vi "Ex_1a.vi"() -> ()   [LabVIEW 2023]
uses:
  <vilib>/platform/TimedLoop/XDataNode/XDataNode.xnode
  <vilib>/Platform/TimedLoop/XDataNode/nitl_modes.ctl
  <vilib>/Platform/TimedLoop/XDataNode/wakeup.ctl
  <vilib>/Platform/TimedLoop/XDataNode/timing_clust.ctl
  <vilib>/DAQmx/create/channels.llb/DAQmx Create Channel (AI-Voltage-Basic).vi
  <vilib>/DAQmx/read.llb/DAQmx Read (Analog DBL 1Chan 1Samp).vi
  <vilib>/Analysis/NI_AALBase.lvlib
  <vilib>/Analysis/baseanly.llb/Mean (DBL).vi
panel:
  out "min":dbl
  out "max":dbl
  out "mean":dbl
  out "Current  Value":dbl
  out "Waveform Graph":dynamicdata(graph)
  in  "Acceleration Unit 2":bool
  out "Current Data Point":dbl
  out "Waveform Chart":dbl(graph)
  in  "?":bool
  in  "?":bool
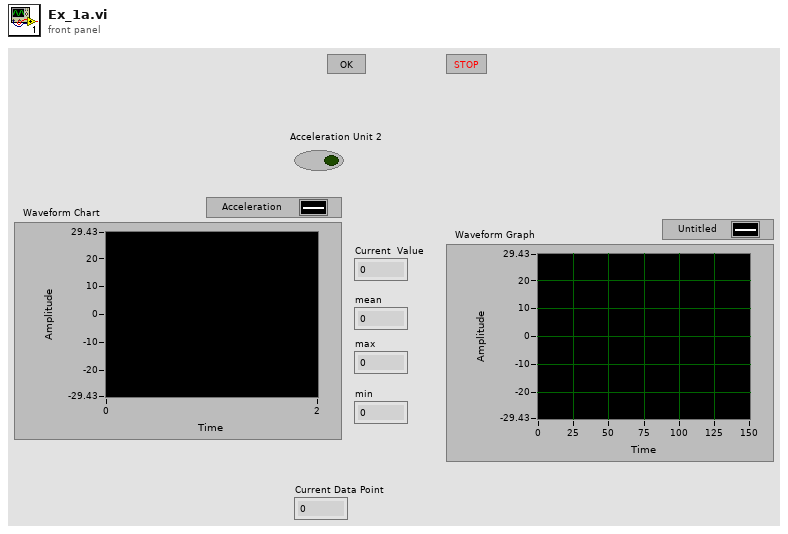
[diagram p1: front panel]
types:
  T1 = typedef "XDNodeRunTimeDep.lvlib/timing_clust.ctl" = cluster{"Expected End [f-1]":u64, "Actual End [f-1]":u64, "Finished Late? [f-1]":bool, "Expected End [i-1]":u64, "Actual End [i-1]":u64, "Finished Late? [i-1]":bool, "Expected Start [i]":u64, "Actual Start [i]":u64, "Expected Start [f]":u64, "Actual Start [f]":u64, "Source Name":string, "Structure Name":string, "Period":i64, "Deadline":i64, "Offset":i64, "Start":i64, "Priority":i32, "Timeout":i32, "Mode":T2, "Wakeup Reason":T3, "Error":errorcluster, "Source Type":string, "Secondary Source Type":string, "Global End Time":u64, "Global Start Time":u64, "Frame Duration":u64, "Iteration Duration":u64, "Assigned CPU":i32, "I/O Scan Engine Mode":u32}
  T2 = typedef "XDNodeRunTimeDep.lvlib/nitl_modes.ctl" = enum32{"No Change", "Process missed periods, maintain original phase", "Discard missed periods, maintain original phase", "Process missed periods, ignore original phase", "Discard missed periods, ignore original phase"}
  T3 = typedef "XDNodeRunTimeDep.lvlib/wakeup.ctl" = enum32{"Normal", "Aborted", "Asynchronous wakeup", "Timing source error", "Timed loop error", "Timeout"}
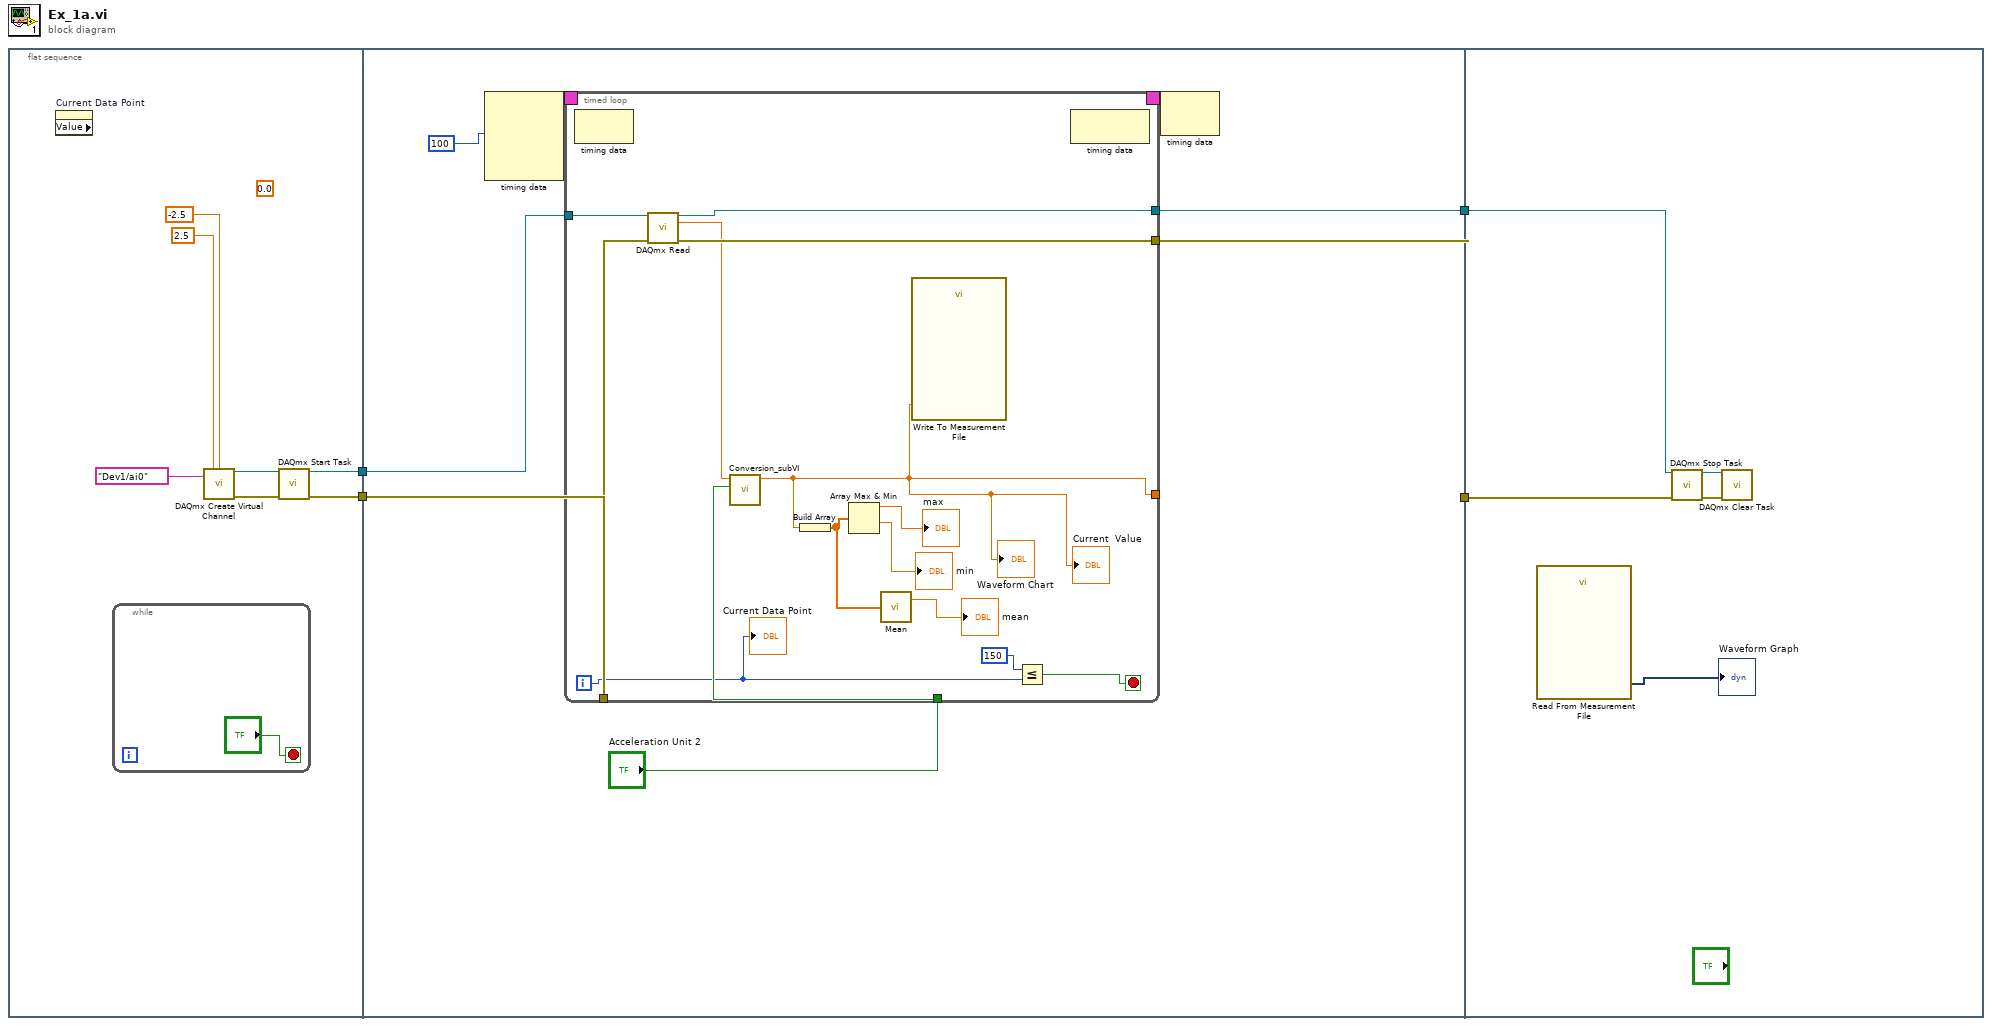
[diagram p0: block diagram]
diagram:
  n1 = flat-sequence {
    tunnel: [w9] -> w4
    tunnel: [w8] -> w2
    tunnel: w4 -> [w16]
    tunnel: [w15] -> w3
    tunnel: w2 -> [w17]
    tunnel: [w13] -> w1
    tunnel: w3 -> [w43]
    tunnel: w1 -> [w42]
    frame #0 {
      (unwired) 0.0
      n2 = property on="Current Data Point" class="DigNum (strict)" props=["Value"]() -> ()  [unwired: 2 in, 3 out]
      n3 = while {
        stop <- "?" stop-if-true
      }
      n4 = call-poly <vilib>:"DAQmx Create Virtual Channel.vi"("maximum value"=2.5, "minimum value"=-2.5, "physical channels"=tag "Dev1/ai0") -> ("task out"=w11:refnum<k21>, "error out"=w10:errorcluster)  [unwired: 11 in]
      n5 = call <vilib>:"DAQmx Start Task.vi"("task/channels in"=w11, "error in"=w10) -> ("task out"=w8:refnum<k21>, "error out"=w9:errorcluster)  [unwired: 12 in]
    }
    frame #1 {
      n6 = node-c288(100) -> (w20:T1)  [unwired: 3 in]
      n7 = timed-loop {
        timing: w20 -> [_]
        timing-out: [_] -> w19
        tunnel: w17 -> [w34]
        tunnel: w16 -> [w33]
        tunnel: [w32] -> w15
        tunnel: "Acceleration Unit 2" -> [w31]
        tunnel: [w30] -> w13
        tunnel: [w25] -> _
        i -> [w26]
        stop <- w27 stop-if-true
        n8 = node-c288() -> ()  [unwired: 1 in, 1 out]
        n9 = call-poly <vilib>:"DAQmx Read.vi"("task/channels in"=w34, "error in"=w33) -> ("task out"=w30:refnum<k21>, "data"=w29:dbl, "error out"=w32:errorcluster)  [unwired: 11 in]
        n10 = call "Conversion_subVI.vi"("Acceleration Unit in"=w31, "data"=w29) -> ("Numeric"=w25:dbl)  [unwired: 9 in]
        "Waveform Chart" <- w25
        "Current  Value" <- w25
        n11 = Build Array(w25) -> (w23:dbl[])
        n12 = Array Max & Min(array=w23) -> (max value=→"max":dbl, min value=→"min":dbl)  [unwired: 2 out]
        n13 = call-poly <vilib>:"Mean.vi"("X"=w23) -> ("mean"=→"mean":dbl)  [unwired: 1 out]
        n14 = call "Write To Measurement File"("Signals"=w25) -> ()  [unwired: 16 in, 3 out]
        n15 = Less Or Equal?(x=150, y=w26) -> (x <= y?=w27:bool)
        n16 = node-c288() -> ()  [unwired: 1 in, 1 out]
        "Current Data Point" <- w26
      }
      n17 = node-c288(w19) -> ()  [unwired: 1 out]
    }
    frame #2 {
      n18 = call "Read From Measurement File"() -> ("Signals"=→"Waveform Graph":dynamicdata)  [unwired: 6 in, 5 out]
      n19 = call <vilib>:"DAQmx Stop Task.vi"("task/channels in"=w42, "error in"=w43) -> ("task out"=w45:refnum<k21>, "error out"=w44:errorcluster)  [unwired: 12 in]
      n20 = call <vilib>:"DAQmx Clear Task.vi"("task in"=w45, "error in"=w44) -> ()  [unwired: 13 in, 1 out]
    }
  }
